vi "Main.vi"(11 "Module Admin":refnum<class "Delacor_lib_QMH_Module Admin.lvclass">) -> ()   [LabVIEW 2019, in "Model.lvlib"]
doc: "This template is based off of the Queued Message Handler design pattern and the Queued Message Handler project template that ships with LabVIEW.\n\nThe main difference is that the queue is private to this module and communication between modules is performed via Broadcast and Request events.\n\nRequest events are wrapped in public API methods and are handled in the Event Handling Loop (EHL) of this VI. Any module can register for Broadcast events sent by this module. The EHL generates messages based on user interface actions.\n\nThe Message Handling Loop (MHL) processes messages generated by the EHL, or by other messages. The messages are string values, so new messages can be added easily to the Message Cases case structure in the MHL. Each message cluster can also provide an optional value for Message Data, which is a variant that can be converted to whatever message-specific data is required.\n_____\nBased on DQMH Project Template 6.0.0.91."
uses:
  Model.lvlib
  <vilib>/Delacor/Delacor QMH/Libraries/Module Admin_class/Delacor_lib_QMH_Module Admin.lvclass
  Module Data--cluster.ctl
  <vilib>/Delacor/Delacor QMH/Libraries/Message Queue_class/Delacor_lib_QMH_Message Queue.lvclass/Delacor_lib_QMH_Message Queue.ctl
  Stop Argument--cluster.ctl
  <vilib>/Delacor/Delacor QMH/Libraries/Module Admin_class/Delacor_lib_QMH_Module Admin.lvclass/Delacor_lib_QMH_Module Admin.ctl
  <vilib>/Utility/miscctls.llb/LVPointTypeDef.ctl
  <vilib>/Delacor/Delacor QMH/Libraries/Message Queue_class/Delacor_lib_QMH_Enqueue Message (Single).vi
  <vilib>/Delacor/Delacor QMH/Libraries/Module Admin_class/Delacor_lib_QMH_Get External Launch.vi
  <vilib>/Utility/error.llb/Error Cluster From Error Code.vi
  <vilib>/ErrorRing/Error Ring.xnode
  <vilib>/Delacor/Delacor QMH/Libraries/Message Queue_class/Delacor_lib_QMH_Message Queue.lvclass
  Controller/Controller.lvlib
panel:
  out "error out":errorcluster
  out "Status":string
  in  "Simulate MHL Error":bool
  in  "Simulate EHL Error":bool
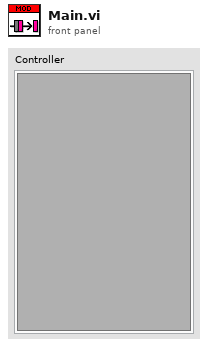
[diagram p1: front panel]
types:
  T1 = typedef "Controller.lvlib/Broadcast Events--cluster.ctl" = cluster{"Module Did Init":refnum<user-event>, "Status Updated":refnum<user-event>, "Error Reported":refnum<user-event>, "Module Did Stop":refnum<user-event>, "Update Module Execution Status":refnum<user-event>}
  T2 = typedef "Model.lvlib/Request Events--cluster.ctl" = cluster{"Stop Module":refnum<user-event>, "Show Panel":refnum<user-event>, "Hide Panel":refnum<user-event>, "Get Module Execution Status":refnum<user-event>, "Show Diagram":refnum<user-event>}
  T3 = typedef "Model.lvlib/Module Data--cluster.ctl" = cluster{"Status":string}
  T4 = enum32{"invalid lock state", "Not Locked", "Locked (No Password)", "Password-protected"}
  T5 = typedef "Model.lvlib/Stop Argument--cluster.ctl" = cluster{"Origin":string, "Exit via Stop Module Req?":bool, "Wait for Module to stop?":bool}
  T6 = typedef "LVPointTypeDef.ctl" = cluster{"Horizontal":i16, "Vertical":i16}
  T7 = enum32{"Invalid", "Standard", "Closed", "Hidden", "Minimized", "Maximized"}
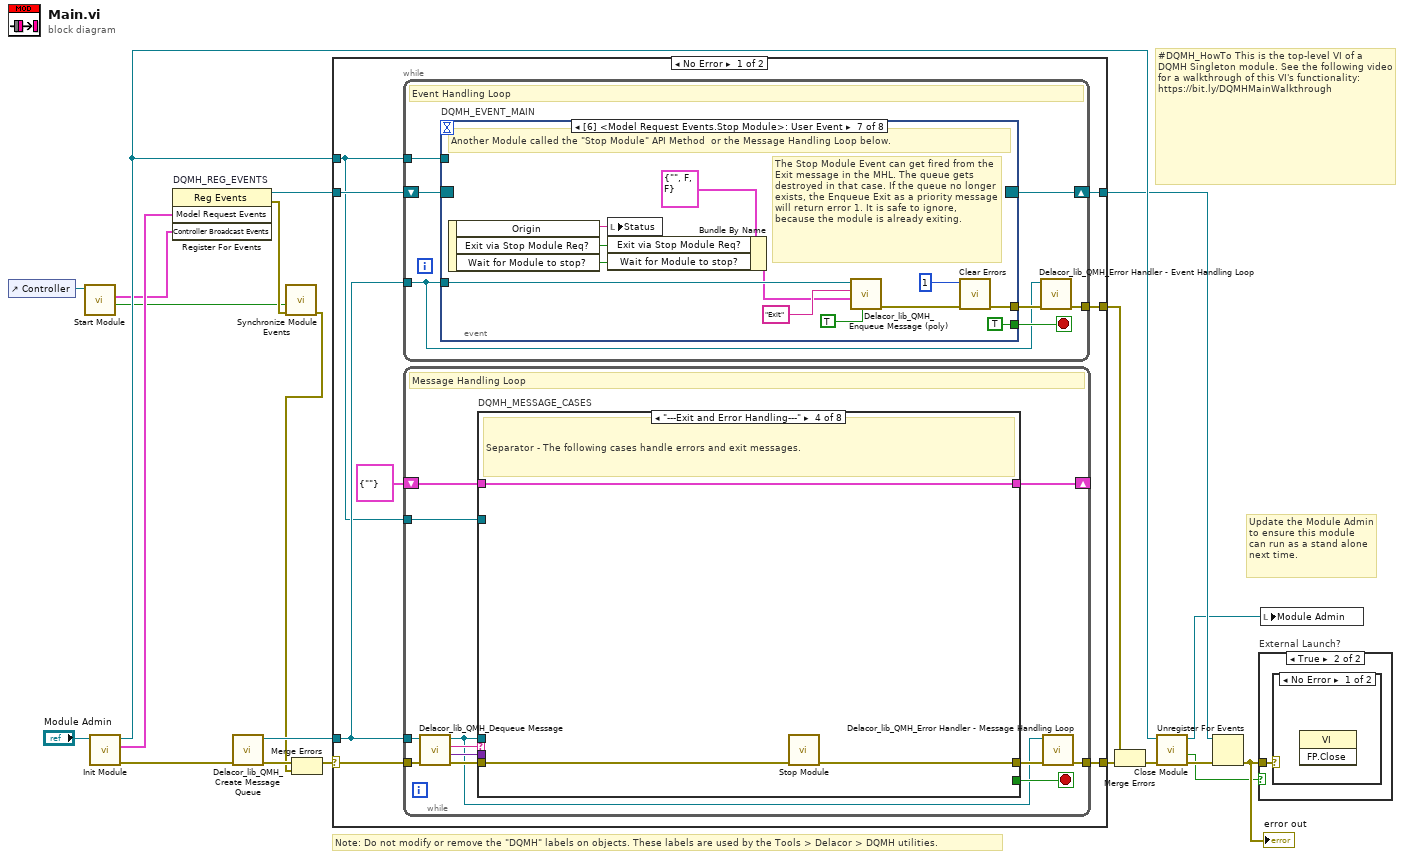
[diagram p0: block diagram]
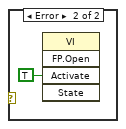
[diagram p3: hidden frame]
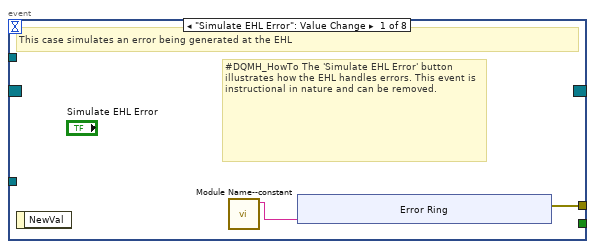
[diagram p4: hidden frame]
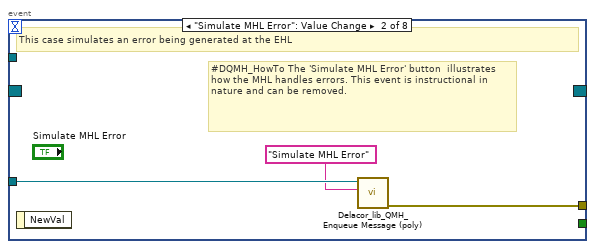
[diagram p5: hidden frame]
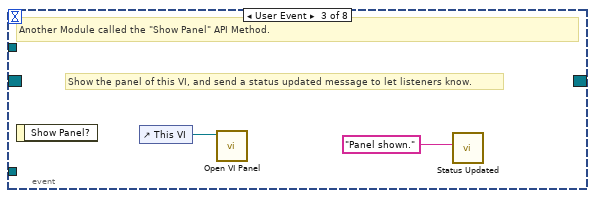
[diagram p6: hidden frame]
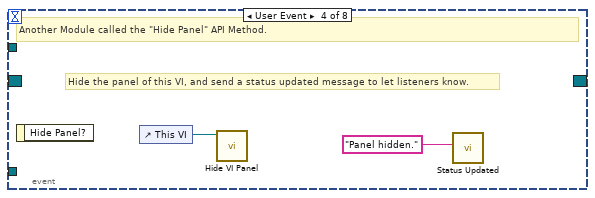
[diagram p7: hidden frame]
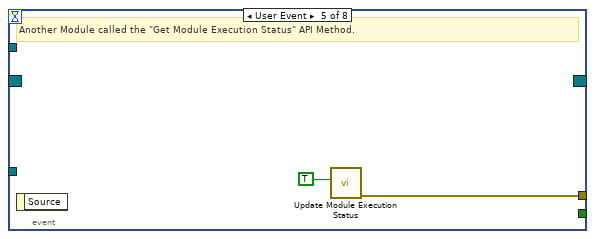
[diagram p8: hidden frame]
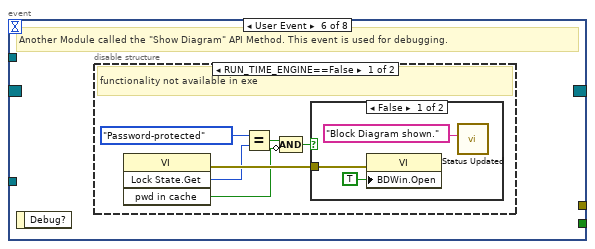
[diagram p9: hidden frame]
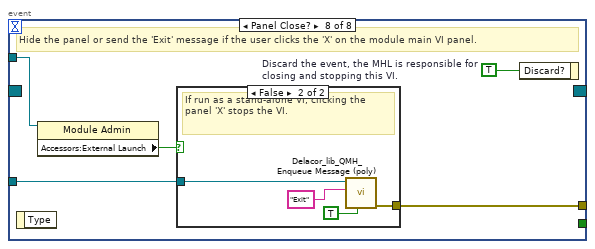
[diagram p12: hidden frame]
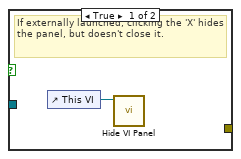
[diagram p13: hidden frame]
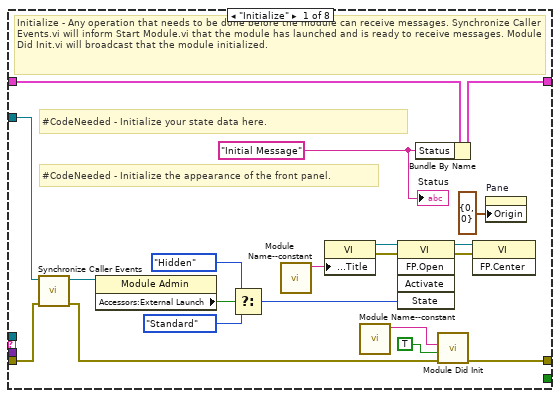
[diagram p14: hidden frame]
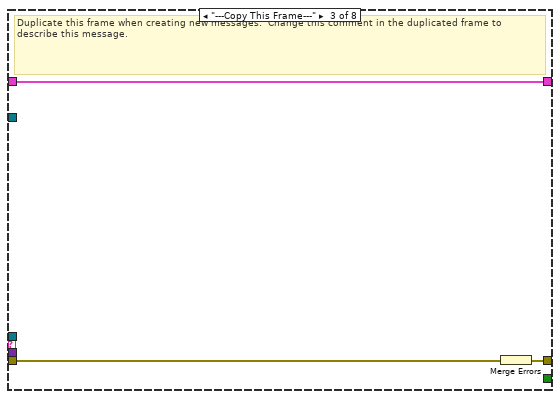
[diagram p16: hidden frame]
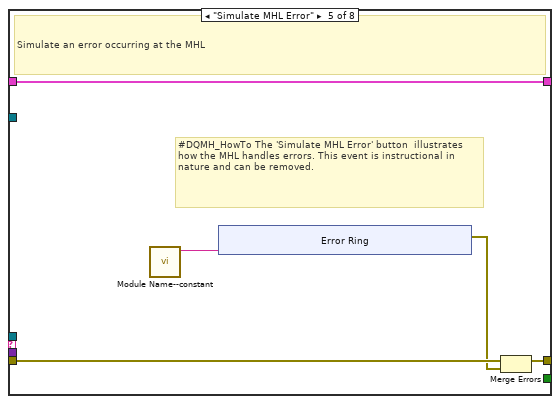
[diagram p17: hidden frame]
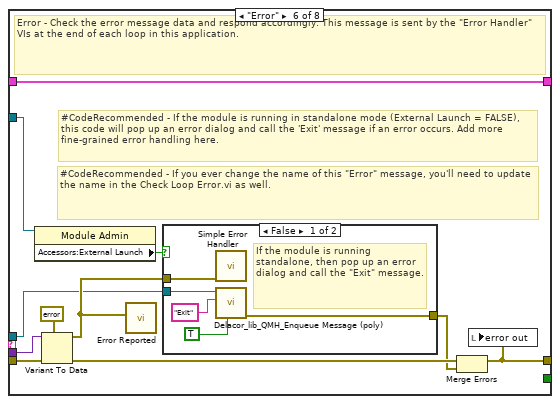
[diagram p18: hidden frame]
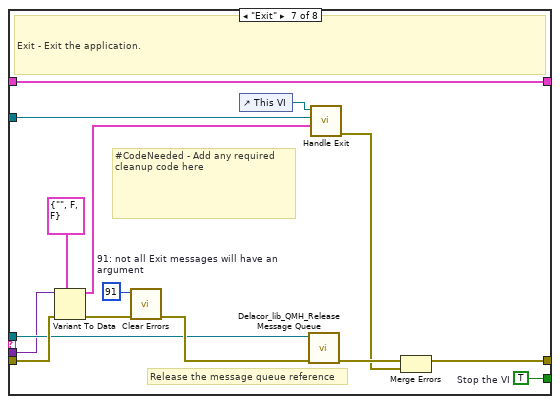
[diagram p20: hidden frame]
diagram:
  # "#DQMH_HowTo This is the top-level VI of a DQMH Singleton module. See the following video for a walkthrough of this VI's functionality: https://bit.ly/DQMHMainWalkthrough"
  # "Note: Do not modify or remove the \"DQMH\" labels on objects. These labels are used by the Tools > Delacor > DQMH utilities."
  # "Update the Module Admin to ensure this module can run as a stand alone next time."
  n1 = control-ref of="Controller"() -> (w5:refnum<vi>)
  n2 = call "Start Module.vi"("Subpanel Ref"=w5) -> ("Wait for Event Sync?"=w2:bool, "Controller Broadcast Events"=w4:T1)  [unwired: 7 in, 2 out]
  n3 = call "Init Module.vi"("Singleton Module Admin in"="Module Admin") -> ("error out"=w20:errorcluster, "Model Request Events"=w10:T2, "Singleton Module Admin out"=w13:refnum<class "Delacor_lib_QMH_Module Admin.lvclass">)  [unwired: 8 in]
  n4 = register-events "DQMH_REG_EVENTS"(w10, w4) -> (reference out=w11:refnum<event-registration>, error out=w3:errorcluster)  [unwired: 2 in]
  n5 = call <vilib>:"Delacor_lib_QMH_Create Message Queue.vi"("error in"=w20) -> ("error out"=w15:errorcluster, "Message Queue"=w9:refnum<class "Delacor_lib_QMH_Message Queue.lvclass">)  [unwired: 9 in]
  n6 = call "Synchronize Module Events.vi"("error in"=w3, "Wait for Event Sync?"=w2) -> ("error out"=w1:errorcluster)  [unwired: 9 in]
  n7 = Merge Errors(w15, w1) -> (w14:errorcluster)
  n8 = case shown="No Error" w14 {
    selector: w14 -> [w27 w185]
    tunnel: [w29 w184] -> w21
    tunnel: [w26 w190] -> w12
    tunnel: w11 -> [w24 w190]
    tunnel: w9 -> [w23 w183]
    tunnel: [w28 _] -> w18
    tunnel: w13 -> [w22 w186]
    frame No Error {
      n9 = while {
        tunnel: w23 -> [w30]
        shift-right: [w33] -> w26
        shift-left: w24 -> [w34]
        tunnel: [w35] -> w28
        tunnel: w22 -> [w31]
        stop <- w32 stop-if-true
        # "Event Handling Loop"
        n10 = event "DQMH_EVENT_MAIN" shown="[6] <Model Request Events.Stop Module>: User Event" {
          selector: w34 -> [_ _ _ _ _ _ _ _]
          dyn-events: [_ _ _ _ _ _ _ _] -> w33
          timeout: _ -> [_ _ _ _ _ _ _ _]
          tunnel: [_ _ _ _ _ _ TRUE ("Discard?") _] -> w32
          tunnel: w30 -> [_ w47 _ _ _ _ w71 w78]
          tunnel: [w38 w48 _ _ w54 _ w74 w80] -> w36
          tunnel: w31 -> [_ _ _ _ _ _ _ w77]
          event "Simulate EHL Error": Value Change {
            # "#DQMH_HowTo The 'Simulate EHL Error' button  illustrates how the EHL handles errors. This event is instructional in nature and can be removed."
            # "This case simulates an error being generated at the EHL"
            n11 = event-data() -> ()  [unwired: 1 in, 1 out]
            n12 = call "Module Name--constant.vi"() -> ("Module Name"=w37:string)  [unwired: 11 in]
            n13 = xnode "Error Ring"("parameter 0"=w37) -> ("error out"=w38:errorcluster)
          }
          event "Simulate MHL Error": Value Change {
            # "#DQMH_HowTo The 'Simulate MHL Error' button  illustrates how the MHL handles errors. This event is instructional in nature and can be removed."
            # "This case simulates an error being generated at the EHL"
            n14 = event-data() -> ()  [unwired: 1 in, 1 out]
            n15 = call-poly <vilib>:"Delacor_lib_QMH_Enqueue Message (poly).vi"("Message"="Simulate MHL Error", "Message Queue in"=w47) -> ("error out"=w48:errorcluster)  [unwired: 8 in, 1 out]
          }
          event User Event {
            # "Show the panel of this VI, and send a status updated message to let listeners know."
            # "Another Module called the \"Show Panel\" API Method."
            n16 = event-data() -> ()  [unwired: 1 in, 1 out]
            n17 = control-ref of="This VI"() -> (w50:refnum<vi>)
            n18 = call "Open VI Panel.vi"("VI"=w50) -> ()  [unwired: 10 in, 1 out]
            n19 = call "Status Updated.vi"("Status"="Panel shown." ("format string")) -> ()  [unwired: 10 in, 1 out]
          }
          event User Event {
            # "Hide the panel of this VI, and send a status updated message to let listeners know."
            # "Another Module called the \"Hide Panel\" API Method."
            n20 = event-data() -> ()  [unwired: 1 in, 1 out]
            n21 = control-ref of="This VI"() -> (w52:refnum<vi>)
            n22 = call "Hide VI Panel.vi"("VI"=w52) -> ()  [unwired: 10 in, 1 out]
            n23 = call "Status Updated.vi"("Status"="Panel hidden." ("format string")) -> ()  [unwired: 10 in, 1 out]
          }
          event User Event {
            # "Another Module called the \"Get Module Execution Status\" API Method."
            n24 = event-data() -> ()  [unwired: 1 in, 1 out]
            n25 = call "Update Module Execution Status.vi"("Running?"=TRUE) -> ("error out"=w54:errorcluster)  [unwired: 10 in]
          }
          event User Event {
            # "Another Module called the \"Show Diagram\" API Method. This event is used for debugging."
            n26 = event-data() -> ()  [unwired: 1 in, 1 out]
            n27 = disable-structure shown="RUN_TIME_ENGINE==False" {
              frame condition #0 (active) {
                # "functionality not available in exe"
                n28 = invoke class="VI" method="Lock State.Get"() -> (error out=w60:errorcluster, "Get Lock State"=w59:T4, "pwd in cache"=w56:bool)  [unwired: 4 in, 1 out]
                n29 = Equal?(x=T4."Password-protected", y=w59) -> (x = y?=w57:bool)
                n30 = Compound Arithmetic op=AND(w57, invert w56) -> (w55:bool)
                n31 = case shown="False" w55 {
                  tunnel: w60 -> [w63 _]
                  frame False {
                    n32 = property class="VI"(error in=w63, "BDWin.Open"=TRUE ("Block Diagram Window:Open")) -> ()  [unwired: 1 in, 2 out]
                    n33 = call "Status Updated.vi"("Status"="Block Diagram shown." ("format string")) -> ()  [unwired: 10 in, 1 out]
                  }
                  frame True {
                    # "Password-protected VI, and the password is not in the cache. Do not show the diagram."
                  }
                }
              }
              frame condition #1 {
              }
            }
          }
          event User Event {
            # "The Stop Module Event can get fired from the Exit message in the MHL. The queue gets destroyed in that case. If the queue no longer exists, the Enqueue Exit as a priority message will return error 1. It is safe to ignore, because the module is already exiting."
            # "Another Module called the \"Stop Module\" API Method  or the Message Handling Loop below."
            n34 = event-data() -> ("Origin"=w70:string, "Exit via Stop Module Req?"=w66:bool, "Wait for Module to stop?"=w65:bool)  [unwired: 1 in]
            n35 = local write "Status"(w70) -> ()
            n36 = Bundle By Name(cluster=T5 {"Origin"="", "Exit via Stop Module Req?"=FALSE, "Wait for Module to stop?"=FALSE} ("Stop Argument"), "Exit via Stop Module Req?"=w66, "Wait for Module to stop?"=w65) -> (w64:T5)
            n37 = call-poly <vilib>:"Delacor_lib_QMH_Enqueue Message (poly).vi"("Priority Message? (F)"=TRUE, "Message Data"=w64, "Message"="Exit", "Message Queue in"=w71) -> ("error out"=w75:errorcluster)  [unwired: 6 in, 1 out]
            n38 = call <vilib>:"Clear Errors.vi"("error in (no error)"=w75, "specific error code to clear (0: all)"=1) -> ("error out"=w74:errorcluster)  [unwired: 4 in, 1 out]
          }
          event Panel Close? {
            w79 = TRUE  # Discard the event, the MHL is responsible for closing and stopping this VI.
            # "Hide the panel or send the 'Exit' message if the user clicks the 'X' on the module main VI panel."
            n39 = event-data() -> ()  [unwired: 1 in, 1 out]
            n40 = property class="Module Admin"(reference=w77) -> ("Accessors:External Launch"=w76:bool)  [unwired: 1 in, 2 out]
            n41 = case shown="False" w76 {
              tunnel: w78 -> [_ w84]
              tunnel: [_ w85] -> w80
              frame True {
                # "If externally launched, clicking the 'X' hides the panel, but doesn't close it."
                n42 = control-ref of="This VI"() -> (w81:refnum<vi>)
                n43 = call "Hide VI Panel.vi"("VI"=w81) -> ()  [unwired: 10 in, 1 out]
              }
              frame False {
                # "If run as a stand-alone VI, clicking the panel 'X' stops the VI."
                n44 = call-poly <vilib>:"Delacor_lib_QMH_Enqueue Message (poly).vi"("Priority Message? (F)"=TRUE, "Message"="Exit", "Message Queue in"=w84) -> ("error out"=w85:errorcluster)  [unwired: 7 in, 1 out]
              }
            }
            n45 = event-data("Discard?"=w79) -> ()  [unwired: 1 in, 1 out]
          }
        }
        n46 = call-dynamic "Delacor_lib_QMH_Error Handler - Event Handling Loop.vi"("error in"=w36, "Message Queue in"=w30) -> ("dup error in"=w35:errorcluster)  [unwired: 8 in, 1 out]
      }
      n47 = while {
        tunnel: w23 -> [w88]
        shift-right: [w92] -> _
        shift-left: T3 {"Status"=""} ("Data Cluster") -> [w93]
        tunnel: w27 -> [w96]
        tunnel: [w94] -> w29
        tunnel: w22 -> [w86]
        stop <- w91 stop-if-true
        # "Message Handling Loop"
        n48 = call-dynamic "Delacor_lib_QMH_Dequeue Message.vi"("error in"=w96, "Message Queue in"=w88) -> ("error out"=w95:errorcluster, "Message Data"=w89:variant, "Message"=w90:string, "Message Queue out"=w87:refnum<class "Delacor_lib_QMH_Message Queue.lvclass">)  [unwired: 6 in]
        n49 = case "DQMH_MESSAGE_CASES" shown="\"---Exit and Error Handling---\"" w90 {
          selector: w90 -> [_ _ _ _ _ _ _ w170]
          tunnel: w87 -> [_ _ _ _ _ w140 w162 _]
          tunnel: w95 -> [w115 w119 w122 w124 w130 w147 w168 w172]
          tunnel: [w113 w119 w121 w123 w129 w143 w165 w173] -> w97
          tunnel: w93 -> [w104 w118 w120 w125 w127 w142 w161 w171]
          tunnel: [w103 w118 w120 w125 w127 w142 w161 w171] -> w92
          tunnel: [_ _ _ _ _ _ w160 _] -> w91
          tunnel: w89 -> [_ _ _ _ _ w141 w159 _]
          tunnel: w86 -> [w105 _ _ _ _ w139 w154 _]
          frame "Initialize" {
            w99 = "Initial Message" ("Initial Message")
            # "#CodeNeeded - Initialize the appearance of the front panel."
            # "#CodeNeeded - Initialize your state data here."
            # "Initialize - Any operation that needs to be done before the module can receive messages. Synchronize Caller Events.vi will inform Start Module.vi that the module has launched and is ready to receive messages. Module Did Init.vi will broadcast that the module initialized."
            n50 = call "Synchronize Caller Events.vi"("error in (no error)"=w115, "Singleton Module Admin in"=w105) -> ("error out"=w114:errorcluster, "Singleton Module Admin out"=w100:refnum<class "Delacor_lib_QMH_Module Admin.lvclass">)  [unwired: 8 in]
            n51 = property class="Module Admin"(reference=w100) -> ("Accessors:External Launch"=w109:bool)  [unwired: 1 in, 2 out]
            n52 = Select(t=T7."Hidden" ("State"), s=w109, f=T7."Standard" ("State")) -> (s? t:f=w106:T7)
            n53 = call "Module Name--constant.vi"() -> ("Module Name"=w112:string)  [unwired: 11 in]
            n54 = property class="VI"("Front Panel.Title"=w112) -> (reference out=w111:refnum<vi>, error out=w117:errorcluster)  [unwired: 2 in]
            n55 = call "Module Name--constant.vi"() -> ("Module Name"=w101:string)  [unwired: 11 in]
            n56 = invoke class="VI" method="FP.Open"(reference=w111, error in=w117, "State"=w106) -> (reference out=w110:refnum<vi>, error out=w116:errorcluster)  [unwired: 2 in, 3 out]
            n57 = Bundle By Name(cluster=w104, "Status"=w99) -> (w103:T3)
            n58 = call "Module Did Init.vi"("error in (no error)"=w114, "Initialized?"=TRUE, "Origin"=w101) -> ("error out"=w113:errorcluster)  [unwired: 8 in]
            n59 = invoke class="VI" method="FP.Center"(reference=w110, error in=w116) -> ()  [unwired: 1 in, 3 out]
            n60 = property on="Pane" class="Pane"("Origin"=T6 {"Horizontal"=0, "Vertical"=0}) -> ()  [unwired: 2 in, 2 out]
            "Status" <- w99
          }
          frame "---Module Specific---" {
            # "Separator -- The following cases handle messages specific to this Module."
          }
          frame "---Copy This Frame---" {
            # "Duplicate this frame when creating new messages.  Change this comment in the duplicated frame to describe this message."
            n61 = Merge Errors(w122) -> (w121:errorcluster)
          }
          frame "---Exit and Error Handling---" {
            # "Separator - The following cases handle errors and exit messages."
            n62 = call "Stop Module.vi"("error in"=w124) -> ("error out"=w123:errorcluster)  [unwired: 10 in]
          }
          frame "Simulate MHL Error" {
            # "#DQMH_HowTo The 'Simulate MHL Error' button  illustrates how the MHL handles errors. This event is instructional in nature and can be removed."
            # "Simulate an error occurring at the MHL"
            n63 = call "Module Name--constant.vi"() -> ("Module Name"=w126:string)  [unwired: 11 in]
            n64 = xnode "Error Ring"("parameter 0"=w126) -> ("error out"=w128:errorcluster)
            n65 = Merge Errors(w130, w128) -> (w129:errorcluster)
          }
          frame "Error" {
            # "#CodeRecommended - If you ever change the name of this \"Error\" message, you'll need to update the name in the Check Loop Error.vi as well."
            # "#CodeRecommended - If the module is running in standalone mode (External Launch = FALSE), this code will pop up an error dialog and call the 'Exit' message if an error occurs. Add more fine-grained error handling here."
            # "Error - Check the error message data and respond accordingly. This message is sent by the \"Error Handler\" VIs at the end of each loop in this application."
            n66 = property class="Module Admin"(reference=w139) -> ("Accessors:External Launch"=w138:bool)  [unwired: 1 in, 2 out]
            n67 = Variant To Data(error in=w147, type=errorcluster {"status"=FALSE, "code"=0, "source"=""} ("error constant"), Variant=w141) -> (data=w148:errorcluster, error out=w145:errorcluster)
            n68 = call "Error Reported.vi"("Error"=w148) -> ()  [unwired: 10 in, 1 out]
            n69 = case shown="False" w138 {
              tunnel: [w153 _] -> w144
              tunnel: w140 -> [w151 _]
              tunnel: w148 -> [w152 _]
              frame False {
                # "If the module is running standalone, then pop up an error dialog and call the \"Exit\" message."
                n70 = call <vilib>:"Simple Error Handler.vi"("error in (no error)"=w152) -> ()  [unwired: 4 in, 5 out]
                n71 = call-poly <vilib>:"Delacor_lib_QMH_Enqueue Message (poly).vi"("Priority Message? (F)"=TRUE, "Message"="Exit", "Message Queue in"=w151) -> ("error out"=w153:errorcluster)  [unwired: 7 in, 1 out]
              }
              frame True {
                # "If the module was launched externally, calling the Error Reported broadcast VI is the only action performed by the \"Error\" message. The module's caller can then process the error appropriately."
              }
            }
            n72 = Merge Errors(w145, w144) -> (w143:errorcluster)
            n73 = local write "error out"(w143) -> ()
          }
          frame "Exit" {
            w158 = 91  # 91: not all Exit messages will have an argument
            w160 = TRUE  # Stop the VI
            # "Release the message queue reference"
            # "#CodeNeeded - Add any required cleanup code here"
            # "Exit - Exit the application."
            n74 = Variant To Data(error in=w168, type=T5 {"Origin"="", "Exit via Stop Module Req?"=FALSE, "Wait for Module to stop?"=FALSE} ("Stop Argument"), Variant=w159) -> (data=w156:T5, error out=w164:errorcluster)
            n75 = call <vilib>:"Clear Errors.vi"("error in (no error)"=w164, "specific error code to clear (0: all)"=w158) -> ("error out"=w167:errorcluster)  [unwired: 4 in, 1 out]
            n76 = control-ref of="This VI"() -> (w155:refnum<vi>)
            n77 = call-dynamic "Delacor_lib_QMH_Release Message Queue.vi"("error in"=w167, "Message Queue"=w162) -> ("error out"=w166:errorcluster)  [unwired: 9 in]
            n78 = call "Handle Exit.vi"("Stop Argument"=w156, "Admin in"=w154, "VI reference"=w155) -> ("error out"=w163:errorcluster)  [unwired: 7 in, 1 out]
            n79 = Merge Errors(w166, w163) -> (w165:errorcluster)
          }
          frame Default {
            # "'Default' case only runs if there is a message that isn't defined in any of the other cases.  Output a programming error."
            n80 = call "Module Name--constant.vi"() -> ("Module Name"=w169:string)  [unwired: 11 in]
            n81 = xnode "Error Ring"("parameter 0"=w170, "parameter 1"=w169) -> ("error out"=w174:errorcluster)
            n82 = Merge Errors(w172, w174) -> (w173:errorcluster)
          }
        }
        n83 = call-dynamic "Delacor_lib_QMH_Error Handler - Message Handling Loop.vi"("error in"=w97, "Message Queue in"=w87) -> ("dup error in"=w94:errorcluster)  [unwired: 8 in, 1 out]
      }
    }
    frame Error {
      # "Synchronize Caller Events.vi will inform Start Module.vi that the module has launched and will let the code calling Start Module.vi register for broadcasts and would permit the caller receive the broadcast that an error occurred at launch time."
      n84 = call-dynamic "Delacor_lib_QMH_Release Message Queue.vi"("error in"=w185, "Message Queue"=w183) -> ("error out"=w184:errorcluster)  [unwired: 9 in]
      n85 = call "Synchronize Caller Events.vi"("Singleton Module Admin in"=w186) -> ("error out"=w191:errorcluster)  [unwired: 9 in, 1 out]
      n86 = call "Module Name--constant.vi"() -> ("Module Name"=w189:string)  [unwired: 11 in]
      n87 = Format Into String(format string="An error occurred during initialization. %s is no longer running.", w189) -> (resulting string=w187:string)  [unwired: 2 in, 1 out]
      n88 = Merge Errors(w184, w191) -> (w192:errorcluster)
      n89 = call "Error Reported.vi"("Additional Information"=w187, "Error"=w192) -> ()  [unwired: 9 in, 1 out]
    }
  }
  n90 = Merge Errors(w18, w21) -> (w17:errorcluster)
  n91 = call "Close Module.vi"("error in (no error)"=w17, "Module Admin in"=w13) -> ("error out"=w19:errorcluster, "External Launch"=w6:bool, "Module Admin out"=w7:refnum<class "Delacor_lib_QMH_Module Admin.lvclass">)  [unwired: 7 in]
  n92 = Unregister For Events(event registration refnum=w12, error in=w19) -> (error out=w16:errorcluster)
  "error out" <- w16
  n93 = case "External Launch?" shown="True" w6 {
    tunnel: w16 -> [_ w193]
    frame False {
    }
    frame True {
      n94 = case shown="No Error" w193 {
        frame No Error {
          n95 = invoke class="VI" method="FP.Close"() -> ()  [unwired: 3 in, 3 out]
        }
        frame Error {
          n96 = invoke class="VI" method="FP.Open"("Activate"=TRUE ("Activate?")) -> ()  [unwired: 4 in, 5 out]
        }
      }
    }
  }
  n97 = local write "Module Admin"(w7) -> ()
